vi "Spindexer_Globals.vi"() -> ()   [LabVIEW 2019]
uses:
  Spindexer_Cluster.ctl
  Spindexer_mode.ctl
panel:
  out "Within Tolerance?":bool
  in  "Spindexer_Set_Notifier":refnum<notifier>
  in  "Spindexer_Execute_Notifier":refnum<notifier>
  in  "Spindexer_Execute_Ref":string="Spindexer_Execute_Ref"
  in  "Spindexer_Set_Ref":string="Spindexer_Set_Ref"
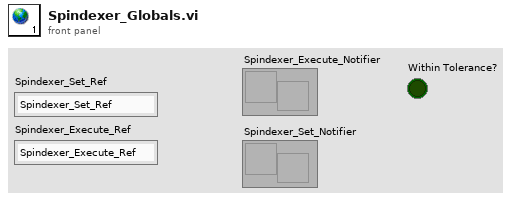
[diagram p1: front panel]
diagram:
